vi "Send SetGlobalThresholdMsg.vi"(8 "error in (no error)":errorcluster, 10 "Threshold":T1=enum."INFO", 11 "Enqueuer in":refnum<class "Message Enqueuer.lvclass">) -> (0 "error out":errorcluster, 3 "Enqueuer out":refnum<class "Message Enqueuer.lvclass">)   [LabVIEW 2026, in "Lumberjack.lvlib" / "SetGlobalThresholdMsg.lvclass"]
uses:
  SetGlobalThresholdMsg.lvclass
  <vilib>/ActorFramework/Message Enqueuer/Message Enqueuer.lvclass
  TypeDefs/Severity.ctl
  SetGlobalThresholdMsg.lvclass/SetGlobalThresholdMsg.ctl
  <vilib>/ActorFramework/Message Enqueuer/Message Enqueuer.lvclass/Message Enqueuer.ctl
  <vilib>/ActorFramework/Message Priority Queue/Priority Enqueue.vi
  Lumberjack.lvlib
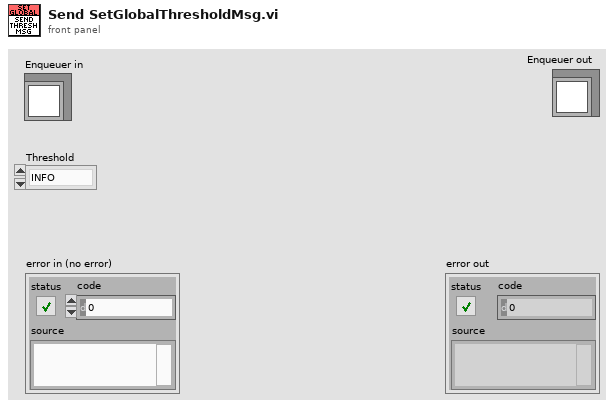
[diagram p1: front panel]
types:
  T1 = typedef "Lumberjack.lvlib/Severity.ctl" = enum16{"OFF", "FATAL", "ERROR", "WARN", "INFO", "DEBUG", "TRACE", "ALL"}
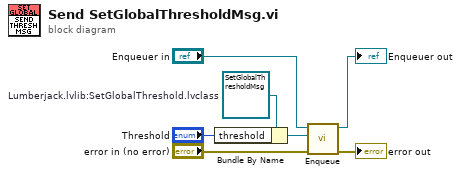
[diagram p0: block diagram]
diagram:
  w3 = refnum<class "SetGlobalThresholdMsg.lvclass"> refnum  # Lumberjack.lvlib:SetGlobalThreshold.lvclass
  n1 = Bundle By Name(cluster=w3, "threshold"="Threshold") -> (w1:refnum<class "SetGlobalThresholdMsg.lvclass">)
  n2 = call <vilib>:"Enqueue.vi"("error in (no error)"="error in (no error)", "Message"=w1, "Message Enqueuer in"="Enqueuer in") -> ("error out"=→"error out":errorcluster, "Message Enqueuer out"=→"Enqueuer out":refnum<class "Message Enqueuer.lvclass">)  [unwired: 7 in]
